vi "add_HeadPan_roslv.vi"(9 "Speed":i32=50, 10 "Units":enum16{"Degrees", "Radians"}(ring), 11 "Pan Angle":sgl) -> (3 "msg out":string)   [LabVIEW 2014]
doc: "Flattens head pan controls into a string"
uses:
  std_msgs/subs/float32Scalar_roslv.vi
  std_msgs/subs/i32Scalar_roslv.vi
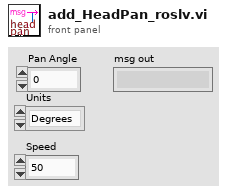
[diagram p1: front panel]
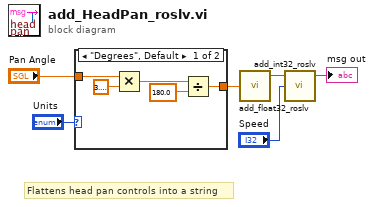
[diagram p0: block diagram]
diagram:
  # "Flattens head pan controls into a string"
  n1 = case shown="\"Degrees\", Default" "Units" {
    tunnel: "Pan Angle" -> [w11 w12]
    tunnel: [w9 w12] -> w1
    frame "Degrees", Default {
      n2 = Multiply(x=w11, y=3.141592653589793) -> (x*y=w10:dbl)
      n3 = Divide(x=w10, y=sgl 180.0) -> (x/y=w9:dbl)
    }
    frame "Radians" {
    }
  }
  n4 = call-poly "add_float32_roslv.vi"("Numeric"=w1) -> ("msg out"=w4:string)  [unwired: 4 in]
  n5 = call-poly "add_int32_roslv.vi"("Numeric"="Speed", "msg in"=w4) -> ("msg out"=→"msg out":string)  [unwired: 3 in]
